vi "Change Settings.vi"(0 "DAQmx Config":T3=[{"Physical channels"="Dev1/ai0", "Channel Name"="pd", "Unit"=0, "Min Voltage"=-1.0, "Max Voltage"=1.0}] {"Unit" items=["Volts", "From Custom Scale"]}, 5 "DAQmx Timing Settings":T2={"rate"=1000.0, "source"="OnboardClock", "sample mode"=10178, "samples per channel"=1000} {"sample mode" items=["Finite Samples"=10178, "Continuous Samples"=10123, "Hardware Timed Single Point"=12522]; "rate" format="%0.2f"}, 7 "Trigger Settings":T1={"Trigger Type"=enum."No Trigger", "Digital Start"={"Source"="", "Digital Start Trigger Edge"=10280}, "Digital Pause"={"Source"="", "Digital Pause Trigger Pause When"=10192}, "Digital Reference"={"Source"="", "Digital Start Trigger Edge"=10280, "Digital Reference Pretrigger Samples"=0}, "Analog Start"={"Source"="", "Analog Slope"=10280, "Analog Start Trigger Hysteresis"=0.0, "Analog Start Trigger Level"=0.0}, "Analog Pause"={"Source"="", "Analog Start Trigger Level"=0.0, "Analog Pause Trigger Pause When"=10093}, "Analog Reference"={"Source"="", "Slope"=10280, "Pretrigger Samples"=0, "Level"=0.0}, "Time Start"={"Select Time\nManually"=FALSE, "When"=timestamp(0 s since 1904-01-01)}} {"Time Start"."When" format="%<%x %.3X>T"; "Analog Reference"."Level" format="%0.2f"; "Analog Reference"."Slope" items=["Rising"=10280, "Falling"=10171]; "Analog Pause"."Analog Pause Trigger Pause When" items=["Above Level"=10093, "Below Level"=10107]; "Analog Pause"."Analog Start Trigger Level" format="%0.2f"; "Analog Start"."Analog Start Trigger Level" format="%0.2f"; "Analog Start"."Analog Start Trigger Hysteresis" format="%.2f"; "Analog Start"."Analog Slope" items=["Rising"=10280, "Falling"=10171]; "Digital Reference"."Digital Start Trigger Edge" items=["Rising"=10280, "Falling"=10171]; "Digital Pause"."Digital Pause Trigger Pause When" items=["High"=10192, "Low"=10214]; "Digital Start"."Digital Start Trigger Edge" items=["Rising"=10280, "Falling"=10171]}, 9 "Calibration Array":cluster{"Slope":dbl, "Offset":dbl}[](array[cluster])=[{"Slope"=1.0, "Offset"=0.0}], 11 "error in (no error)":errorcluster) -> (15 "error out":errorcluster)   [LabVIEW 2020, in "Acquisition.lvlib"]
doc: "Fire an event to change the hardware settings in the helper loop.\n\nThis is a private request event that should only be fired from within the Acquisition Module. If this request was public, other modules could call it and the Settings Editor would not get the notification that the values changed.\n\n_____\nCreated using Delacor QMH Event Scripter 4.0.0.68.\n_____\nBased on DQMH Project Template 6.0.0.91."
uses:
  Acquisition.lvlib
  Settings Editor/DAQmx Config--cluster.ctl
  Settings Editor/DAQmx Timing--cluster.ctl
  Settings Editor/DAQmx Trigger Settings--cluster.ctl
  Settings Editor/Settings Editor.lvlib
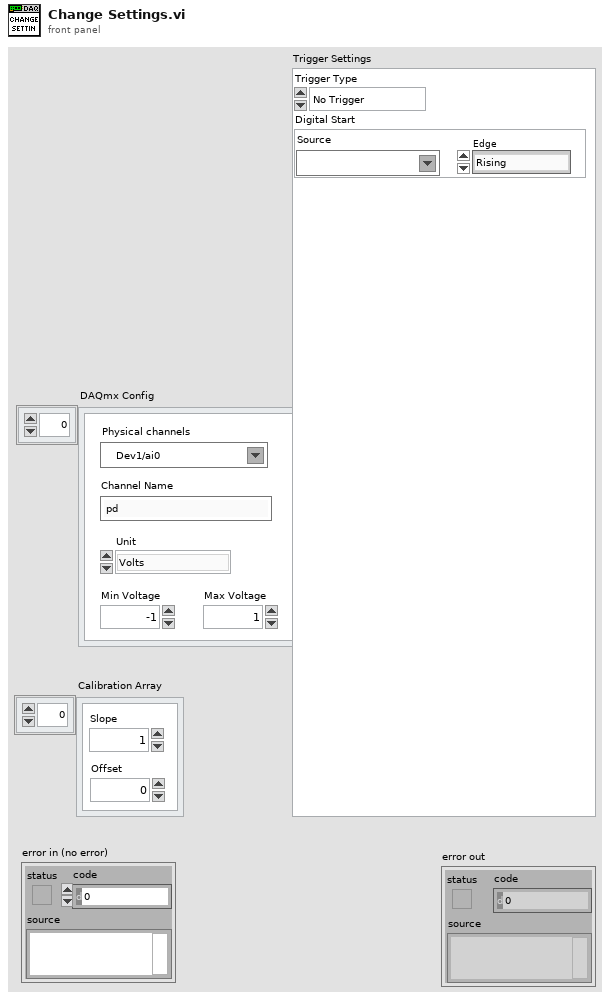
[diagram p1: front panel]
types:
  T1 = typedef "Settings Editor.lvlib/DAQmx Trigger Settings--cluster.ctl" = cluster{"Trigger Type":enum32{"No Trigger", "Digital Start", "Digital Pause", "Digital Reference", "Analog Start", "Analog Pause", "Analog Reference", "Time Start"}, "Digital Start":cluster{"Source":tag, "Digital Start Trigger Edge":i32}, "Digital Pause":cluster{"Source":tag, "Digital Pause Trigger Pause When":i32}, "Digital Reference":cluster{"Source":tag, "Digital Start Trigger Edge":i32, "Digital Reference Pretrigger Samples":u32}, "Analog Start":cluster{"Source":string, "Analog Slope":i32, "Analog Start Trigger Hysteresis":dbl, "Analog Start Trigger Level":dbl}, "Analog Pause":cluster{"Source":string, "Analog Start Trigger Level":dbl, "Analog Pause Trigger Pause When":i32}, "Analog Reference":cluster{"Source":string, "Slope":i32, "Pretrigger Samples":u32, "Level":dbl}, "Time Start":cluster{"Select Time\nManually":bool, "When":timestamp}}
  T2 = typedef "Settings Editor.lvlib/DAQmx Timing--cluster.ctl" = cluster{"rate":dbl, "source":tag, "sample mode":i32, "samples per channel":i32}
  T3 = typedef "Settings Editor.lvlib/DAQmx Config--cluster.ctl" = cluster{"Physical channels":tag, "Channel Name":string, "Unit":i32, "Min Voltage":dbl, "Max Voltage":dbl}[]
  T4 = cluster{"Calibration Array":cluster{"Slope":dbl, "Offset":dbl}[], "DAQmx Config":T3, "DAQmx Timing Settings":T2, "Trigger Settings":T1}
  T5 = typedef "Acquisition.lvlib/Request Events--cluster.ctl" = cluster{"Stop Module":refnum<user-event>, "Show Panel":refnum<user-event>, "Hide Panel":refnum<user-event>, "Get Module Execution Status":refnum<user-event>, "Show Diagram":refnum<user-event>, "Stop Acquiring":refnum<user-event>, "Wakeup Helper Loop":refnum<user-event>, "Change Settings":refnum<user-event>, "Calibrate DAQ":refnum<user-event>, "Start Acquiring":refnum<user-event>}
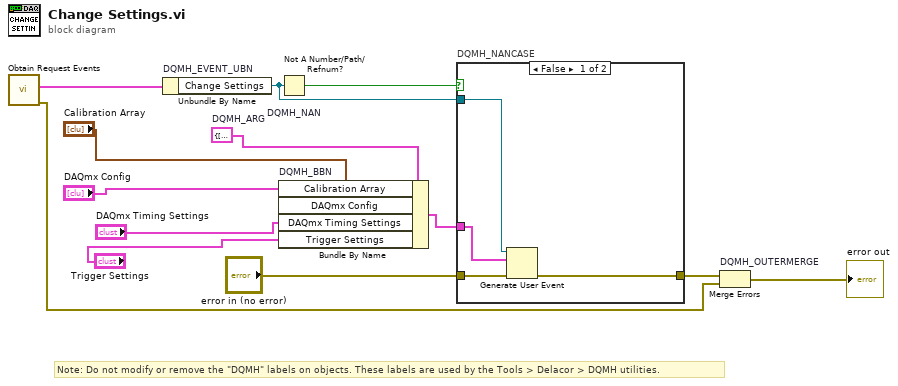
[diagram p0: block diagram]
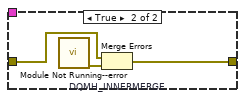
[diagram p2: hidden frame]
diagram:
  w5 = T4 {"Calibration Array"=[{"Slope"=1.0, "Offset"=0.0}], "DAQmx Config"=[{"Physical channels"="Dev1/ai0", "Channel Name"="pd", "Unit"=0, "Min Voltage"=-1.0, "Max Voltage"=1.0}], "DAQmx Timing Settings"={"rate"=1000.0, "source"="OnboardClock", "sample mode"=10178, "samples per channel"=1000}, "Trigger Settings"={"Trigger Type"=enum."No Trigger", "Digital Start"={"Source"="", "Digital Start Trigger Edge"=10280}, "Digital Pause"={"Source"="", "Digital Pause Trigger Pause When"=10192}, "Digital Reference"={"Source"="", "Digital Start Trigger Edge"=10280, "Digital Reference Pretrigger Samples"=0}, "Analog Start"={"Source"="", "Analog Slope"=10280, "Analog Start Trigger Hysteresis"=0.0, "Analog Start Trigger Level"=0.0}, "Analog Pause"={"Source"="", "Analog Start Trigger Level"=0.0, "Analog Pause Trigger Pause When"=10093}, "Analog Reference"={"Source"="", "Slope"=10280, "Pretrigger Samples"=0, "Level"=0.0}, "Time Start"={"Select Time\nManually"=FALSE, "When"=timestamp(0 s since 1904-01-01)}}}  # DQMH_ARG
  # "Note: Do not modify or remove the \"DQMH\" labels on objects. These labels are used by the Tools > Delacor > DQMH utilities."
  n1 = call "Obtain Request Events.vi"() -> ("error out"=w7:errorcluster, "Acquisition Request Events"=w6:T5)  [unwired: 10 in]
  n2 = Unbundle By Name "DQMH_EVENT_UBN"(w6) -> ("Change Settings"=w9:refnum<user-event>)
  n3 = Not A Number/Path/Refnum? "DQMH_NAN"(number/path/refnum=w9) -> (NaN/Path/Refnum?=w10:bool)
  n4 = Bundle By Name "DQMH_BBN"(cluster=w5, "Calibration Array"="Calibration Array", "DAQmx Config"="DAQmx Config", "DAQmx Timing Settings"="DAQmx Timing Settings", "Trigger Settings"="Trigger Settings") -> (w11:T4)
  n5 = case "DQMH_NANCASE" shown="False" w10 {
    tunnel: "error in (no error)" -> [w17 w20]
    tunnel: [w16 w19] -> w8
    tunnel: w9 -> [w15 _]
    tunnel: w11 -> [w14 _]
    frame False {
      n6 = Generate User Event(user event=w15, event data cluster=w14, error in=w17) -> (error out=w16:errorcluster)  [unwired: 1 in, 1 out]
    }
    frame True {
      n7 = call "Module Not Running--error.vi"() -> ("error out"=w18:errorcluster)  [unwired: 11 in]
      n8 = Merge Errors "DQMH_INNERMERGE"(w20, w18) -> (w19:errorcluster)
    }
  }
  n9 = Merge Errors "DQMH_OUTERMERGE"(w8, w7) -> (→"error out":errorcluster)
